vi "rename channel.vi"(8 "error in":errorcluster, 9 "new name":string, 10 "old name":string, 11 "CVT configuration in":refnum<class "CVT configuration.lvclass">) -> (0 "error out":errorcluster, 3 "CVT configuration out":refnum<class "CVT configuration.lvclass">)   [LabVIEW 2013, in "CVT configuration.lvclass"]
uses:
  CVT configuration.lvclass
  CVT configuration.lvclass/CVT configuration.ctl
  <vilib>/NI/Tag Bus/tag/tag descriptor.lvclass/tag descriptor.ctl
  <vilib>/NI/Tag Bus/tag/read tag name.vi
  <vilib>/NI/Tag Bus/tag/tag descriptor.lvclass
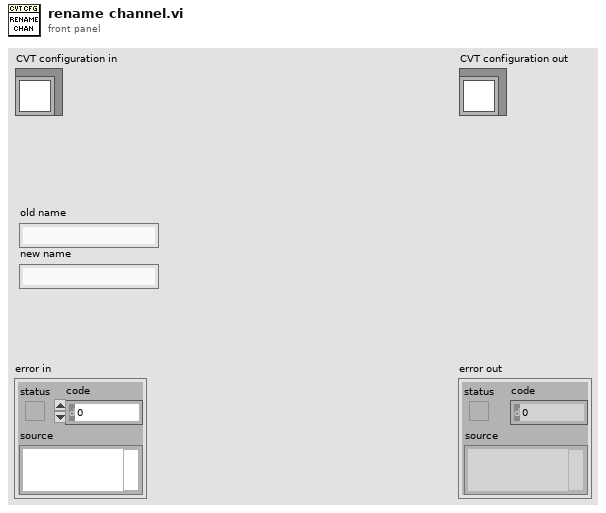
[diagram p1: front panel]
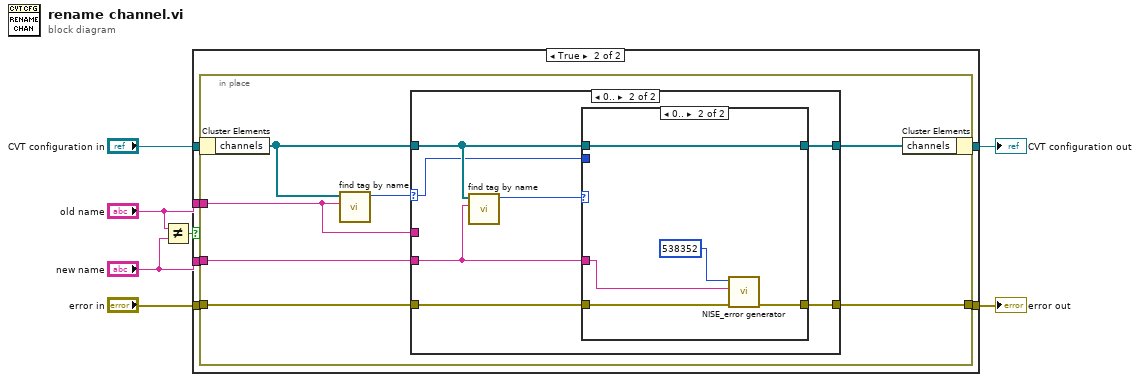
[diagram p0: block diagram]
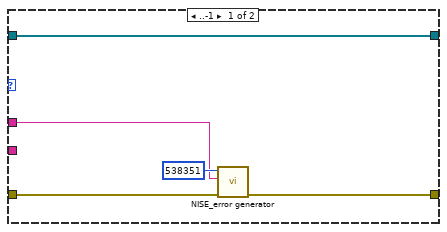
[diagram p3: hidden frame]
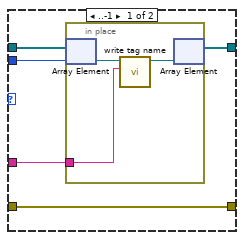
[diagram p4: hidden frame]
diagram:
  n1 = Not Equal?(x="old name", y="new name") -> (x != y?=w3:bool)
  n2 = case shown="True" w3 {
    tunnel: "error in" -> [w8 w15]
    tunnel: "CVT configuration in" -> [w9 w14]
    tunnel: [w9 w13] -> w5
    tunnel: [w8 w12] -> w4
    tunnel: "new name" -> [_ w11]
    tunnel: "old name" -> [_ w10]
    frame False {
    }
    frame True {
      n3 = in-place {
        in-place-border: w11 -> [w18]
        in-place-border: [w21] -> w12
        in-place-border: w15 -> [w19]
        in-place-border: w10 -> [w16]
        n4 = in-place-cluster #1(w14) -> ("channels"=w22:refnum<class "TBM channel.lvclass">[])
        n5 = call <vilib>:"find tag by name.vi"("name"=w16, "tags in"=w22) -> ("index"=w17:i32)  [unwired: 9 in]
        n6 = case shown="0.." w17 {
          selector: w17 -> [_ w28]
          tunnel: w22 -> [w24 w33]
          tunnel: w16 -> [w26 _]
          tunnel: [w25 w29] -> w21
          tunnel: [w24 w34] -> w20
          tunnel: w19 -> [w23 w30]
          tunnel: w18 -> [_ w32]
          frame ..-1 {
            n7 = call <vilib>:"NISE_error generator.vi"("error in"=w23, "append error message"=w26, "error code (0)"=538351) -> ("error out"=w25:errorcluster)  [unwired: 6 in]
          }
          frame 0.. {
            n8 = call <vilib>:"find tag by name.vi"("name"=w32, "tags in"=w33) -> ("index"=w31:i32)  [unwired: 9 in]
            n9 = case shown="0.." w31 {
              tunnel: [w39 w47] -> w34
              tunnel: w28 -> [w38 _]
              tunnel: w33 -> [w37 w47]
              tunnel: w32 -> [w36 w43]
              tunnel: w30 -> [w35 w45]
              tunnel: [w35 w46] -> w29
              frame ..-1 {
                n10 = in-place {
                  in-place-border: w36 -> [w40]
                  n11 = in-place-array #2(w37, w38) -> (w42:refnum<class "TBM channel.lvclass">)
                  n12 = call <vilib>:"write tag name.vi"("name"=w40, "system tag in"=w42) -> ("system tag out"=w41:refnum<class "TBM channel.lvclass">)  [unwired: 8 in, 1 out]
                  n13 = in-place-array #2(w41) -> (w39:refnum<class "TBM channel.lvclass">[])  [unwired: 1 out]
                }
              }
              frame 0.. {
                n14 = call <vilib>:"NISE_error generator.vi"("error in"=w45, "append error message"=w43, "error code (0)"=538352) -> ("error out"=w46:errorcluster)  [unwired: 6 in]
              }
            }
          }
        }
        n15 = in-place-cluster #1("channels"=w20) -> (w13:refnum<class "CVT configuration.lvclass">)
      }
    }
  }
  "error out" <- w4
  "CVT configuration out" <- w5
